vi "PH_SHS_Analysis_Calibrator.destructor.vi"(0 "i ref in":refnum<vi>, 5 "error in(no error)":errorcluster) -> (19 "error out":errorcluster)   [LabVIEW 2014, in "PH_SHS_Analysis_Calibrator.lvlib"]
doc: "This is the destructor of a class.\n\nLicense Agreement for this software:\n\nCopyright (C)\nGesellschaft für Schwerionenforschung, GSI\nPlanckstr. 1\n64291 Darmstadt\nGermany\n\nContact: D.Beck@gsi.de \n\nThis program is free software; you can redistribute it and/or modify it under the terms of the \nGNU General Public License as published by the Free Software Foundation; either version 2 of \nthe license, or (at your option) any later version.\n\nThis program is distributed in the hope that it will be useful, but WITHOUT ANY WARRANTY; \nwithout even the implied warranty of MERCHANTABILITY or FITNESS FOR A PARTICULAR PURPOSE. See the GNU General License for more details (http://www.gnu.org).\n\nGesellschaft für Schwerionenforschung, GSI\nPlanckstr. 1, 64291 Darmstadt, Germany\nFor all questions and ideas contact: M.Richter@gsi.de, H.Brand@gsi.de or D.Beck@gsi.de.\nLast update: 16-JUN-2004"
uses:
  PH_SHS_Analysis_Calibrator.lvlib
  PH_Basics/PH_Img_BaseClass/PH_Img_BaseClass.lvlib
  PH_Basics/PH_SM_Class/PH_SM_Class.lvlib
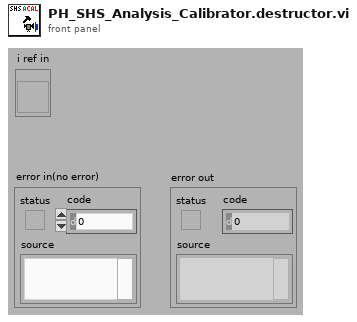
[diagram p1: front panel]
types:
  T1 = enum16{"SetAttribute", "GetAttribute", "CreateAttribute", "DestroyAttribute", "DestroyAllAtributes"}
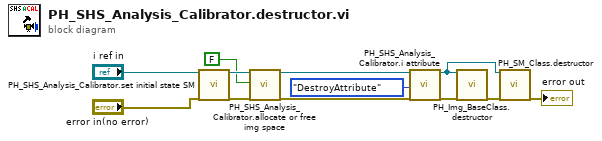
[diagram p0: block diagram]
diagram:
  n1 = call "PH_SHS_Analysis_Calibrator.set initial state SM.vi"("i ref in"="i ref in", "error in (no error)"="error in(no error)") -> ("i ref out"=w9:refnum<vi>, "error out"=w11:errorcluster)  [unwired: 16 in]
  n2 = call "PH_SHS_Analysis_Calibrator.allocate or free img space.vi"("i ref in"=w9, "Allocate?"=FALSE ("Create?"), "error in (no error)"=w11) -> ("i ref out"=w8:refnum<vi>, "error out"=w10:errorcluster)  [unwired: 15 in]
  n3 = call "PH_SHS_Analysis_Calibrator.i attribute.vi"("VI Refnum"=w8, "Action"=T1."DestroyAttribute", "error in (no error)"=w10) -> ("VI Refnum out"=w2:refnum<vi>, "error out"=w1:errorcluster)  [unwired: 14 in, 1 out]
  n4 = call "PH_Img_BaseClass.destructor.vi"("i ref in"=w2, "error in(no error)"=w1) -> ("error out"=w4:errorcluster)  [unwired: 17 in]
  n5 = call "PH_SM_Class.destructor.vi"("i ref in"=w2, "error in(no error)"=w4) -> ("error out"=→"error out":errorcluster)  [unwired: 17 in]
